vi "Get VIRef from Library.vi"(8 "error in (no error)":errorcluster, 10 "item name":string, 11 "library in":refnum<vi>) -> (0 "error out":errorcluster, 1 "found":bool, 2 "vi":refnum<vi>, 3 "library out":refnum<vi>)   [LabVIEW 2019, in "gRPC Template Creation Utility.lvlib"]
uses:
  gRPC Template Creation Utility.lvlib
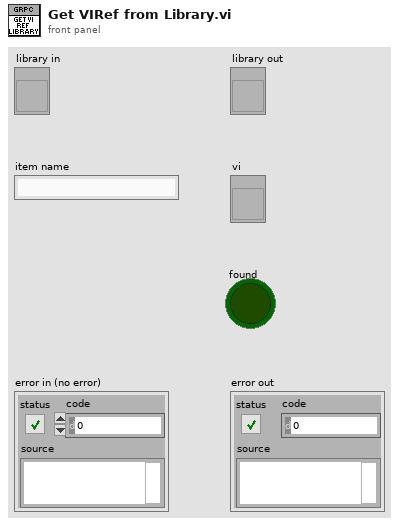
[diagram p1: front panel]
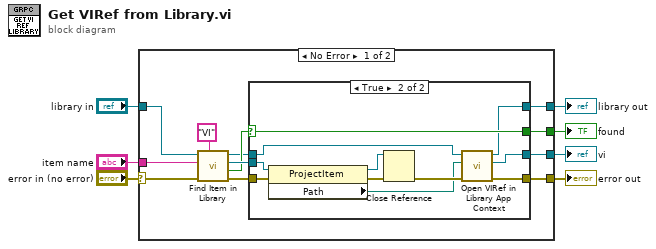
[diagram p0: block diagram]
diagram:
  n1 = case shown="No Error" "error in (no error)" {
    selector: "error in (no error)" -> [w13 w34]
    tunnel: "library in" -> [w17 w35]
    tunnel: "item name" -> [w15 _]
    tunnel: [w8 w35] -> w5
    tunnel: [w14 w34] -> w4
    tunnel: [w11 _] -> w2
    tunnel: [w10 _] -> w1
    frame No Error {
      n2 = call "Find Item in Library.vi"("Item Type"="VI", "error in (no error)"=w13, "Item Name"=w15, "Library item in"=w17) -> ("error out"=w19:errorcluster, "Found?"=w12:bool, "Project Item (Library Item)"=w18:refnum<vi>, "Library item out"=w9:refnum<vi>)  [unwired: 4 in]
      n3 = case shown="True" w12 {
        selector: w12 -> [w21 w31]
        tunnel: w19 -> [w22 w33]
        tunnel: w18 -> [_ w32]
        tunnel: [w22 w23] -> w14
        tunnel: [w21 w31] -> w11
        tunnel: [_ w24] -> w10
        tunnel: w9 -> [w20 w27]
        tunnel: [w20 w26] -> w8
        frame False {
        }
        frame True {
          n4 = property class="ProjectItem"(reference=w32, error in=w33) -> (reference out=w29:refnum<vi>, error out=w30:errorcluster, "Path"=w25:path)
          n5 = Close Reference(reference=w29, error in (no error)=w30) -> (error out=w28:errorcluster)
          n6 = call "Open VIRef in Library App Context.vi"("error in (no error)"=w28, "vi path"=w25, "library in"=w27) -> ("error out"=w23:errorcluster, "vi"=w24:refnum<vi>, "library out"=w26:refnum<vi>)  [unwired: 6 in]
        }
      }
    }
    frame Error {
    }
  }
  "library out" <- w5
  "error out" <- w4
  "found" <- w2
  "vi" <- w1
